vi "write TBM configuration.vi"(8 "error in":errorcluster, 10 "configuration":refnum<class "TBM configuration.lvclass">, 11 "fixed module parent implementation editor node in":refnum<class "fixed channel editor.lvclass">) -> (0 "error out":errorcluster, 3 "fixed module parent implementation editor node out":refnum<class "fixed channel editor.lvclass">)   [LabVIEW 2013, in "fixed channel editor.lvclass"]
uses:
  fixed channel editor.lvclass
  <vilib>/NI/Tag Bus Module Framework/root configuration/TBM configuration.lvclass
  <vilib>/NI/Configuration Framework/NISE_CEF_TreeControl.lvlib
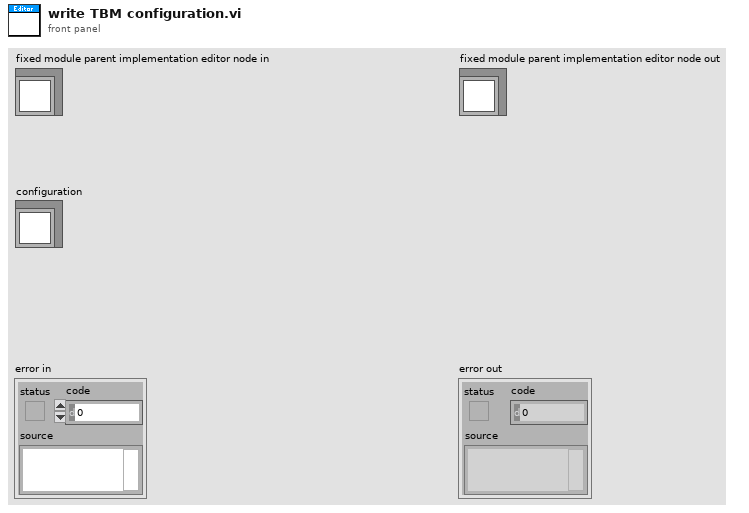
[diagram p1: front panel]
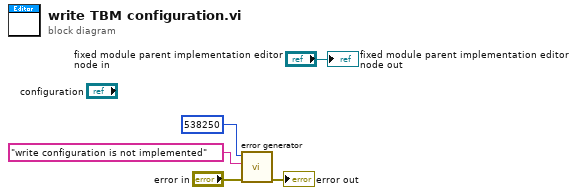
[diagram p0: block diagram]
diagram:
  n1 = call <vilib>:"error generator.vi"("error in"="error in", "append error message"="write configuration is not implemented", "error code (0)"=538250) -> ("error out"=→"error out":errorcluster)  [unwired: 6 in]
  "fixed module parent implementation editor node out" <- "fixed module parent implementation editor node in"
